vi "checkCached.vi"(10 "Old":refnum<class "URI.lvclass">, 11 "New URI":refnum<class "URI.lvclass">) -> (3 "URI":refnum<class "URI.lvclass">)   [LabVIEW 2013, in "openURI.lvlib" / "URI.lvclass"]
uses:
  URI.lvclass
  URI.lvclass/URI.ctl
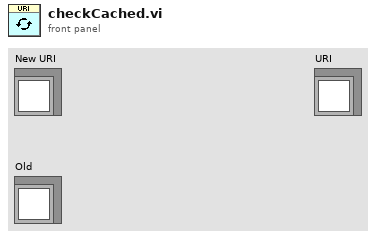
[diagram p1: front panel]
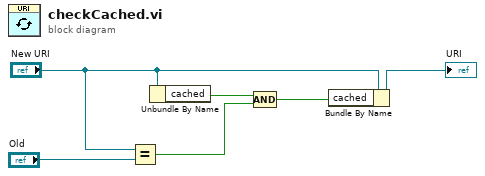
[diagram p0: block diagram]
diagram:
  n1 = Equal?(x="New URI", y="Old") -> (x = y?=w2:bool)
  n2 = Unbundle By Name("New URI") -> ("cached"=w3:bool)
  n3 = Compound Arithmetic op=AND(w3, w2) -> (w1:bool)
  n4 = Bundle By Name(cluster="New URI", "cached"=w1) -> (→"URI":refnum<class "URI.lvclass">)
